vi "Expression Breaker.vi"(11 "result string":string) -> (3 "Array":string[](array[string]))   [LabVIEW 2014]
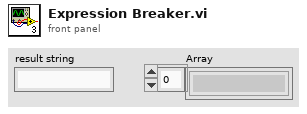
[diagram p1: front panel]
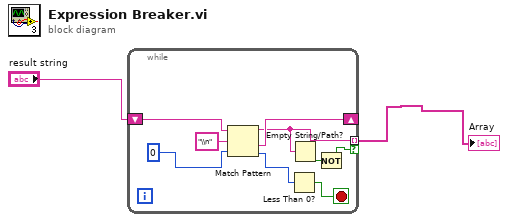
[diagram p0: block diagram]
diagram:
  n1 = while {
    shift-right: [w9] -> _
    shift-left: "result string" -> [w10]
    tunnel: [w5] -> w2 mode=indexing if=w3
    stop <- w8 stop-if-true
    n2 = Match Pattern(string=w10, regular expression="\\n", offset (0)=0 ("offset past match")) -> (before substring=w5:string, after substring=w9:string, offset past match=w7:i32)  [unwired: 1 out]
    n3 = Less Than 0?(x=w7) -> (x < 0?=w8:bool)
    n4 = Empty String/Path?(string/path=w5) -> (empty?=w4:bool)
    n5 = Not(x=w4) -> (.not. x?=w3:bool)
  }
  "Array" <- w2
